vi "CubeLiftSubsystem.vi"   [LabVIEW 2017]
uses:
  Subsystem/Subsystem.lvclass
  CubeLiftCommand.ctl
  SubsystemData/CubeLiftData/CubeLiftData.lvclass
  <vilib>/Rock Robotics/WPI/ThirdParty/Phoenix-LabVIEW/Motor Controller/Controls/CTRE_Phoenix_MotorControl_ControlMode.ctl
  CubeLiftOutput.ctl
panel:
  # "This is responsable for controling the lifts"
types:
  T1 = typedef "CubeLiftData.lvclass/CubeLiftOutput.ctl" = cluster{"LiftOutputSetting":dbl, "DepositCube?":bool, "LiftControlMode":T2}
  T2 = typedef "CTRE_Phoenix_MotorControl_ControlMode.ctl" = u16
  T3 = typedef "CubeLiftData.lvclass/CubeLiftCommand.ctl" = cluster{"Bucket":cluster{"Deposit":bool}, "Slide":cluster{"Slide command":enum16{"Up", "Down", "Stationary"}}}
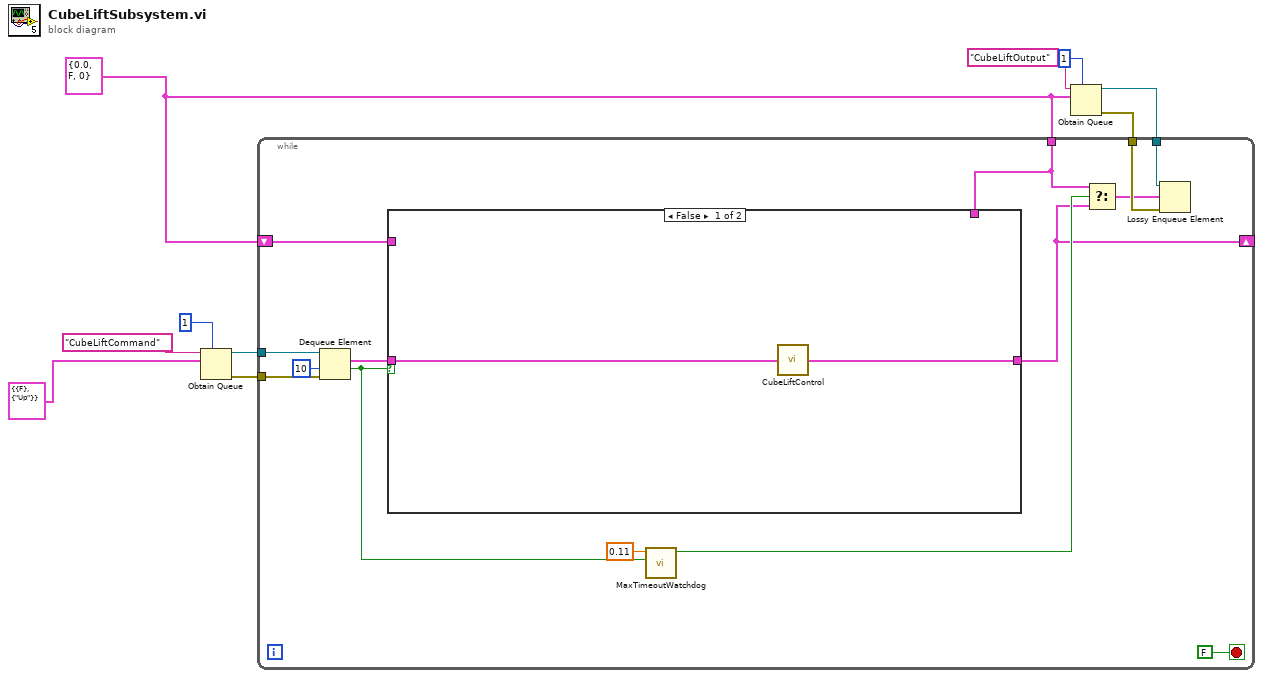
[diagram p0: block diagram]
diagram:
  w4 = T1 {"LiftOutputSetting"=0.0, "DepositCube?"=FALSE, "LiftControlMode"=0} ("CubeLiftOutput")
  n1 = Obtain Queue(max queue size (-1, unlimited)=1, name (unnamed)="CubeLiftCommand", element data type=T3 {"Bucket"={"Deposit"=FALSE}, "Slide"={"Slide command"=enum."Up"}} ("Cube Lift Command")) -> (queue out=w8:refnum<queue>, error out=w7:errorcluster)  [unwired: 2 in, 1 out]
  n2 = Obtain Queue(max queue size (-1, unlimited)=1, name (unnamed)="CubeLiftOutput", element data type=w4) -> (queue out=w2:refnum<queue>, error out=w3:errorcluster)  [unwired: 2 in, 1 out]
  n3 = while {
    tunnel: w8 -> [w23]
    tunnel: w7 -> [w22]
    shift-right: [w11] -> _
    shift-left: w4 -> [w13]
    tunnel: w4 -> [w14]
    tunnel: w3 -> [w16]
    tunnel: w2 -> [w17]
    stop <- FALSE stop-if-true
    n4 = Dequeue Element(queue=w23, timeout in ms (-1)=10, error in (no error)=w22) -> (element=w18:T3, timed out?=w20:bool)  [unwired: 2 out]
    n5 = case shown="False" w20 {
      tunnel: w18 -> [w26 _]
      tunnel: w14 -> [_ _]
      tunnel: w13 -> [_ w27]
      tunnel: [w25 w27] -> w11
      frame False {
        n6 = call "CubeLiftControl.vi"("Cube Lift Command"=w26) -> ("CubeLiftOutput"=w25:T1)  [unwired: 6 in]
      }
      frame True {
      }
    }
    n7 = call "MaxTimeoutWatchdog.vi"("Keep counting?"=w20, "Max Timeout (s)"=0.11 ("Time Target (s)")) -> ("Over Max Timeout?"=w15:bool)  [unwired: 9 in]
    n8 = Select(t=w14, s=w15, f=w11) -> (s? t:f=w12:T1)
    n9 = Lossy Enqueue Element(queue=w17, element=w12, error in (no error)=w16) -> ()  [unwired: 4 out]
  }
